vi "MagSpecAnalyzeSingleImage.vi"(4 "empty image":bool, 6 "Cluster in":T6, 7 "Camera Settings":T2, 9 "2D":T1, 10 "One time calculation":T3, 11 "Refnum in":T5) -> (1 "Cluster out":cluster{dbl[][]}, 2 "Boolean":bool, 3 "spec cluster 2":cluster{"Momentum [MeV/C]":dbl[], dbl[]}, 5 "time: 2Dinter":u32)   [LabVIEW 2020, in "MagSpec_Bella.lvclass"]
uses:
  MagSpec_Bella.lvclass
  finalCalib--Cluster.ctl
  IMAQ Image.ctl
  OneTimeCalculation.ctl
  OnOffTypeDef.ctl
  CameraSettings_File.ctl
  2D.ctl
  CamAndObj_TypDEf_Bella.ctl
  ScreenCam2_TypDEf_Bella.ctl
  NI_Vision_Development_Module.lvlib
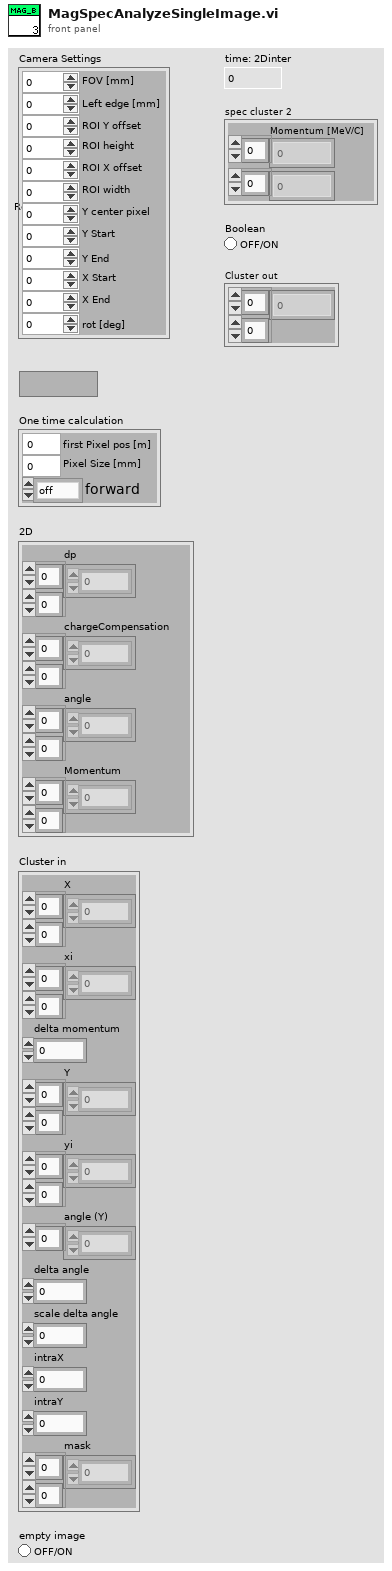
[diagram p1: front panel]
types:
  T1 = typedef "2D.ctl" = cluster{"dp":dbl[][], "chargeCompensation":dbl[][], "angle":dbl[][], "Momentum":dbl[][]}
  T2 = typedef "CameraSettings_File.ctl" = cluster{"FOV [mm]":dbl, "Left edge [mm]":dbl, "ROI Y offset":dbl, "ROI height":dbl, "ROI X offset":dbl, "ROI width":dbl, "Y center pixel":dbl, "Y Start":dbl, "Y End":dbl, "X Start":dbl, "X End":dbl, "rot [deg]":dbl}
  T3 = typedef "OneTimeCalculation.ctl" = cluster{"first Pixel pos [m]":dbl, "Pixel Size [mm]":dbl, "forward":T4}
  T4 = typedef "OnOffTypeDef.ctl" = enum16{"off", "on"}
  T5 = typedef "IMAQ Image.ctl" = refnum<image>
  T6 = typedef "finalCalib--Cluster.ctl" = cluster{"X":dbl[][], "xi":dbl[][], "delta momentum":dbl, "Y":dbl[][], "yi":dbl[][], "angle (Y)":dbl[], "delta angle":dbl, "scale delta angle":dbl, "intraX":dbl, "intraY":dbl, "mask":dbl[][]}
  T7 = cluster{"npix-X":i32, "npix-Y":i32, "Left [pix]":dbl, "Top [pix]":dbl}
  T8 = typedef "ScreenCam2_TypDEf_Bella.ctl" = cluster{"Screen Orientation":string, "Screen angle":string, "Lens":T9, "Calibration (mm/pix)":dbl}
  T9 = typedef "CamAndObj_TypDEf_Bella.ctl" = enum16{"FL1-f8x08", "FL1-f8x06", "FL1-f8", "ch300-f50", "FL2G-f8", "FL3M14-f8", "FL3M14-f8x08", "FL3M14-f8x08(2x2)"}
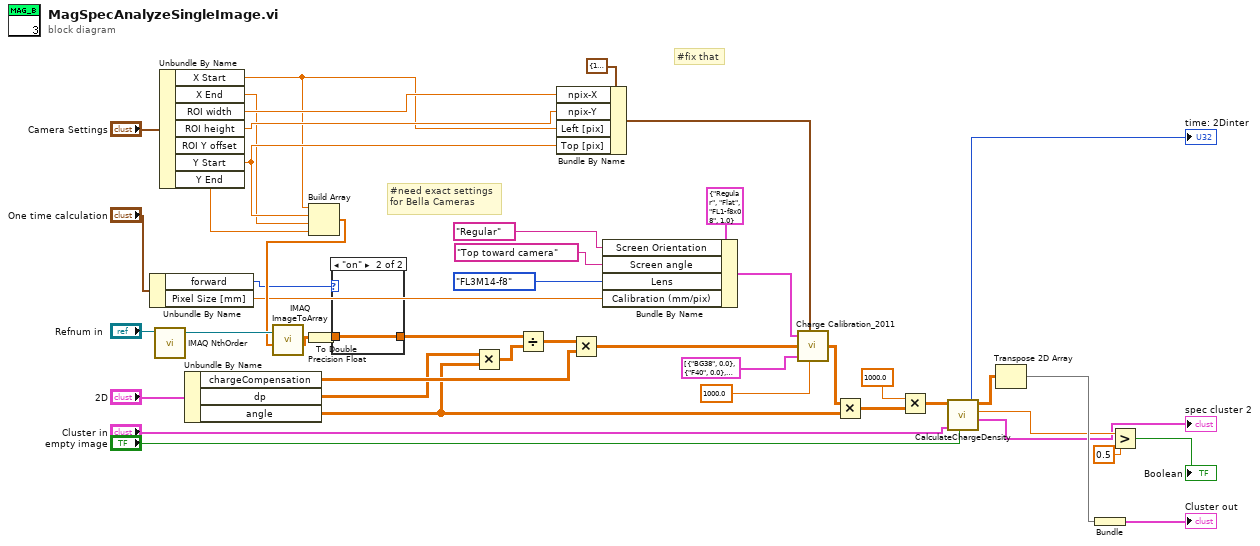
[diagram p0: block diagram]
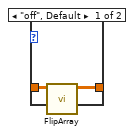
[diagram p2: hidden frame]
diagram:
  # "#fix that"
  # "#need exact settings\nfor Bella Cameras"
  n1 = Unbundle By Name("One time calculation") -> ("forward"=w29:T4, "Pixel Size [mm]"=w5:dbl)
  n2 = call "IMAQ NthOrder"("Image Src"="Refnum in") -> ("Image Dst Out"=w31:T5)  [unwired: 6 in, 1 out]
  n3 = Unbundle By Name("Camera Settings") -> ("X Start"=w25:dbl, "X End"=w20:dbl, "ROI width"=w27:dbl, "ROI height"=w28:dbl, "Y Start"=w26:dbl, "Y End"=w21:dbl)  [unwired: 1 out]
  n4 = Unbundle By Name("2D") -> ("chargeCompensation"=w18:dbl[][], "dp"=w17:dbl[][], "angle"=w2:dbl[][])
  n5 = Build Array(w25, w26, w20, w21) -> (w30:dbl[])
  n6 = call "IMAQ ImageToArray"("Optional Rectangle"=w30, "Image"=w31) -> ("Image Pixels (Float)"=w35:sgl[][])  [unwired: 2 in, 4 out]
  n7 = To Double Precision Float(number=w35) -> (double precision float=w23:dbl[][])
  n8 = case shown="\"on\"" w29 {
    tunnel: w23 -> [w48 w49]
    tunnel: [w47 w49] -> w24
    frame "off", Default {
      n9 = call "FlipArray.vi"("In"=w48) -> ("Out"=w47:dbl[][])  [unwired: 10 in]
    }
    frame "on" {
    }
  }
  n10 = Multiply(x=w17, y=w2) -> (x*y=w40:dbl[][])
  n11 = Divide(x=w24, y=w40) -> (x/y=w41:dbl[][])
  n12 = Bundle By Name(cluster=T7 {"npix-X"=1384, "npix-Y"=300, "Left [pix]"=0.0, "Top [pix]"=0.0} ("ROI infos"), "npix-X"=w27, "npix-Y"=w28, "Left [pix]"=w25, "Top [pix]"=w26) -> (w34:T7)
  n13 = Multiply(x=w41, y=w18) -> (x*y=w19:dbl[][])
  n14 = Bundle By Name(cluster=T8 {"Screen Orientation"="Regular", "Screen angle"="Flat", "Lens"=enum."FL1-f8x08", "Calibration (mm/pix)"=1.0} ("Screen&Camera 2"), "Screen Orientation"="Regular", "Screen angle"="Top toward camera", "Lens"=CamAndObj_TypDEf_Bella."FL3M14-f8", "Calibration (mm/pix)"=w5) -> (w10:T8)
  n15 = call "Charge Calibration_2011.vi"("Screen&Camera 2"=w10, "ROI infos"=w34, "Image (Counts)"=w19, "Filters"=cluster{"Name":string, "#Filters":dbl}[] [{"Name"="BG38", "#Filters"=0.0}, {"Name"="F40", "#Filters"=0.0}, {"Name"="F70", "#Filters"=1.0}, {"Name"="oldBP", "#Filters"=0.0}], "Electron energy (MeV)"=1000.0) -> ("Image (pC)"=w12:dbl[][])  [unwired: 4 in]
  n16 = Multiply(x=w12, y=w2) -> (x*y=w32:dbl[][])
  n17 = Multiply(x=1000.0, y=w32) -> (x*y=w44:dbl[][])
  n18 = call "CalculateChargeDensity.vi"("empty image"="empty image", "Final"="Cluster in", "Z"=w44) -> ("spec cluster 2"=→"spec cluster 2":cluster{"Momentum [MeV/C]":dbl[], dbl[]}, "charge (sum)"=w38:dbl, "charge density"=w14:dbl[][], "time: 2Dinter"=→"time: 2Dinter":u32)  [unwired: 4 in, 1 out]
  n19 = Transpose 2D Array(2D array=w14) -> (transposed array=w46:dbl[][])
  n20 = Bundle(w46) -> (→"Cluster out":cluster{dbl[][]})  [unwired: 1 in]
  n21 = Greater?(x=w38, y=0.5 ("change threshold")) -> (0:→"Boolean":bool)
